vi "Poly Create.vi"   [LabVIEW 2019, in "Scripting API.lvlib"]
uses:
  Scripting API.lvlib
  Addon/Support Libraries/Protocols.lvlibp
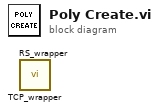
[diagram p0: block diagram]
diagram:
  n1 = call "TCP_wrapper.vi"() -> ()  [unwired: 12 in]
  n2 = call "RS_wrapper.vi"() -> ()  [unwired: 12 in]
